vi "Set Parameters.vi"(8 "error in (no error)":errorcluster, 10 "Parameters":T1, 11 "Execution in":refnum<class "Execution.lvclass">) -> (0 "error out":errorcluster, 3 "Execution out":refnum<class "Execution.lvclass">)   [LabVIEW 2019, in "HTS.lvlib" / "Execution.lvclass"]
uses:
  Execution.lvclass
  VariableContainer/VariableContainer.lvclass
  VariableContainer/Typedefs/Session Handle.ctl
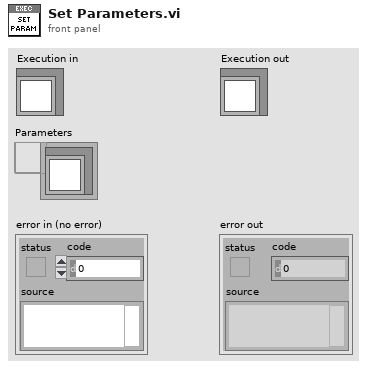
[diagram p1: front panel]
types:
  T1 = typedef "HTS.lvlib/VariableContainer.lvclass/Session Handle.ctl" = refnum<data-value>
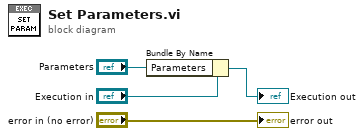
[diagram p0: block diagram]
diagram:
  n1 = Bundle By Name(cluster="Execution in", "Parameters"="Parameters") -> (→"Execution out":refnum<class "Execution.lvclass">)
  "error out" <- "error in (no error)"
